vi "Control Board - Write.vi"(8 "error in (no error)":errorcluster, 9 "LED Outputs":T2, 10 "PWM Outputs":T1, 11 "VISA resource name in":refnum<visa-resource-name>) -> (0 "error out":errorcluster, 3 "VISA resource name out":refnum<visa-resource-name>)   [LabVIEW 2015]
uses:
  LED_Output_TypeDef.ctl
  PWM_Output_TypeDef.ctl
  Inline CRC/CRC SubVIs/Wrappers/CRC-8-Maxim 1-Wire (DOW).vi
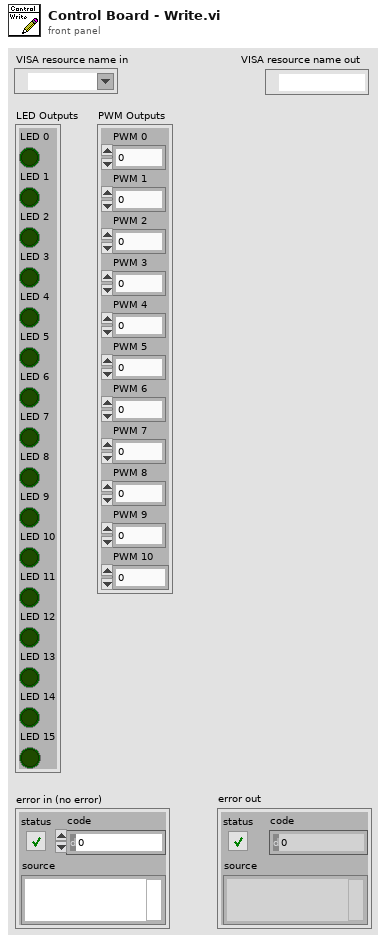
[diagram p1: front panel]
types:
  T1 = typedef "PWM_Output_TypeDef.ctl" = cluster{"PWM 0":u8, "PWM 1":u8, "PWM 2":u8, "PWM 3":u8, "PWM 4":u8, "PWM 5":u8, "PWM 6":u8, "PWM 7":u8, "PWM 8":u8, "PWM 9":u8, "PWM 10":u8}
  T2 = typedef "LED_Output_TypeDef.ctl" = cluster{"LED 0":bool, "LED 1":bool, "LED 2":bool, "LED 3":bool, "LED 4":bool, "LED 5":bool, "LED 6":bool, "LED 7":bool, "LED 8":bool, "LED 9":bool, "LED 10":bool, "LED 11":bool, "LED 12":bool, "LED 13":bool, "LED 14":bool, "LED 15":bool}
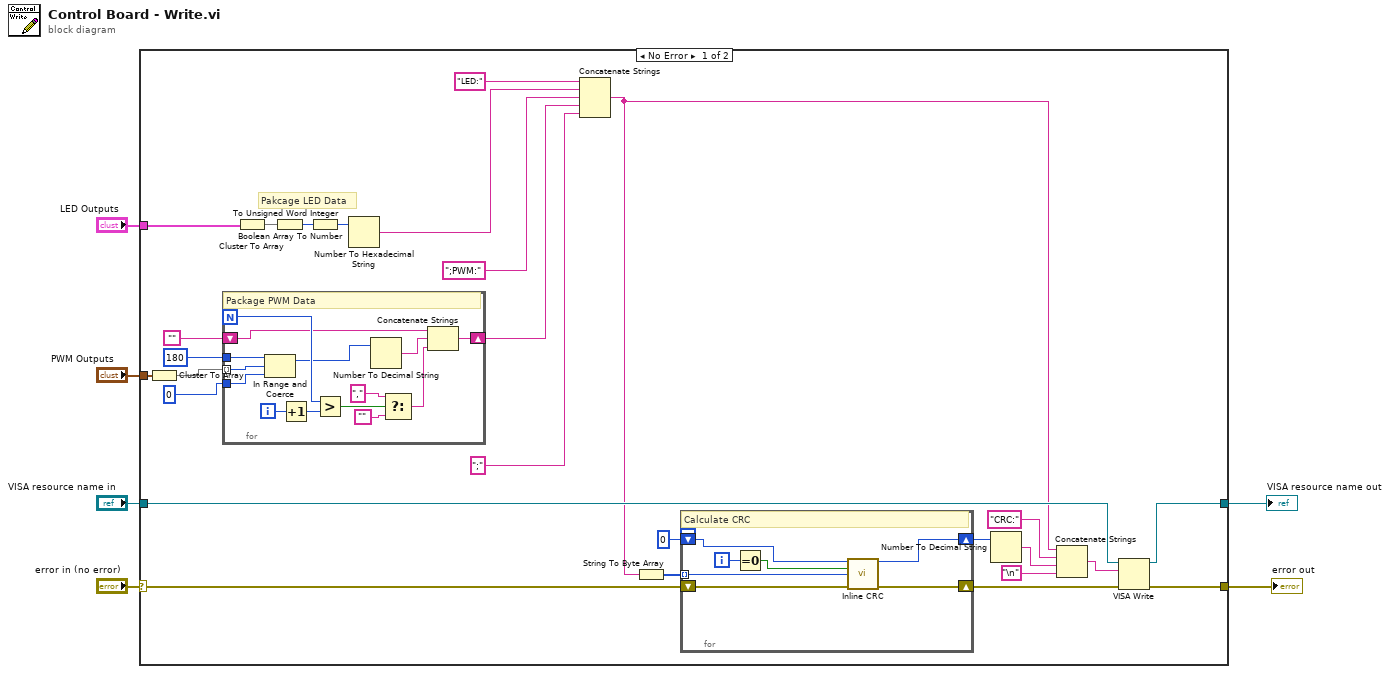
[diagram p0: block diagram]
diagram:
  n1 = case shown="No Error" "error in (no error)" {
    selector: "error in (no error)" -> [w13 w56]
    tunnel: "LED Outputs" -> [w21 _]
    tunnel: "PWM Outputs" -> [w20 _]
    tunnel: [w7 w56] -> w4
    tunnel: "VISA resource name in" -> [w18 w55]
    tunnel: [w8 w55] -> w2
    frame No Error {
      # "Pakcage LED Data"
      n2 = Cluster To Array(cluster=w20) -> (array=w22:u8[])
      n3 = for {
        N -> [w53]
        tunnel: w22 -> [w44] mode=indexing
        shift-right: [w47] -> w28
        shift-left: "" -> [w48]
        tunnel: u8 0 ("upper limit") -> [w42]
        tunnel: u8 180 ("upper limit") -> [w41]
        i -> [w51]
        # "Package PWM Data"
        n4 = In Range and Coerce(upper limit=w41, x=w44, lower limit=w42) -> (coerced(x)=w43:u8)  [unwired: 1 out]
        n5 = Increment(x=w51) -> (x+1=w52:i32)
        n6 = Greater?(x=w53, y=w52) -> (0:w50:bool)
        n7 = Number To Decimal String(number=w43) -> (decimal integer string=w54:string)  [unwired: 1 in]
        n8 = Select(t=",", s=w50, f="") -> (s? t:f=w49:string)
        n9 = Concatenate Strings(w48, w54, w49) -> (w47:string)
      }
      n10 = Cluster To Array(cluster=w21) -> (array=w12:bool[])
      n11 = Boolean Array To Number(Boolean array=w12) -> (number=w11:u32)
      n12 = To Unsigned Word Integer(number=w11) -> (unsigned 16bit integer=w10:u16)
      n13 = Number To Hexadecimal String(2:w10) -> (0:w9:string)  [unwired: 1 in]
      n14 = Concatenate Strings("LED:" ("string"), w9, ";PWM:" ("string"), w28, ";" ("string")) -> (w16:string)
      n15 = String To Byte Array(string=w16) -> (unsigned byte array=w29:u8[])
      n16 = for {
        tunnel: w29 -> [w40] mode=indexing
        shift-right: [w38] -> w31
        shift-left: u8 0 ("CRC In") -> [w39]
        shift-right: [w36] -> w19
        shift-left: w13 -> [w37]
        i -> [w35]
        # "Calculate CRC"
        n17 = Equal To 0?(x=w35) -> (x = 0?=w34:bool)
        n18 = call-poly "Inline CRC.vi"("CRC In"=w39, "Reset"=w34, "Data"=w40, "error in (no error)"=w37) -> ("CRC"=w38:u8, "error out"=w36:errorcluster)  [unwired: 10 in]
      }
      n19 = Number To Decimal String(number=w31) -> (decimal integer string=w32:string)  [unwired: 1 in]
      n20 = Concatenate Strings(w16, "CRC:" ("string"), w32, "\n") -> (w14:string)
      n21 = VISA Write(VISA resource name=w18, write buffer=w14, error in (no error)=w19) -> (VISA resource name out=w8:refnum<visa-resource-name>, error out=w7:errorcluster)  [unwired: 1 out]
    }
    frame Error {
    }
  }
  "error out" <- w4
  "VISA resource name out" <- w2
